vi "plot current.vi"() -> ()   [LabVIEW 2018]
uses:
  <vilib>/Utility/file.llb/Read Delimited Spreadsheet (string).vi
panel:
  out "Run, Subrun":i32[][](array[numeric])
  in  "Card.Channel":dbl=8.04
  in  "End":cluster{"Run":i32, "Subrun":i32}={"Run"=310, "Subrun"=-1}
  in  "Start":cluster{"Run":i32, "Subrun":i32}={"Run"=280, "Subrun"=0}
  out "Timestamp Array":timestamp[](array[timestamp])
  out "Plot":cluster{timestamp[], dbl[]}[](graph)
  # "channel must have 2 significant figures!"
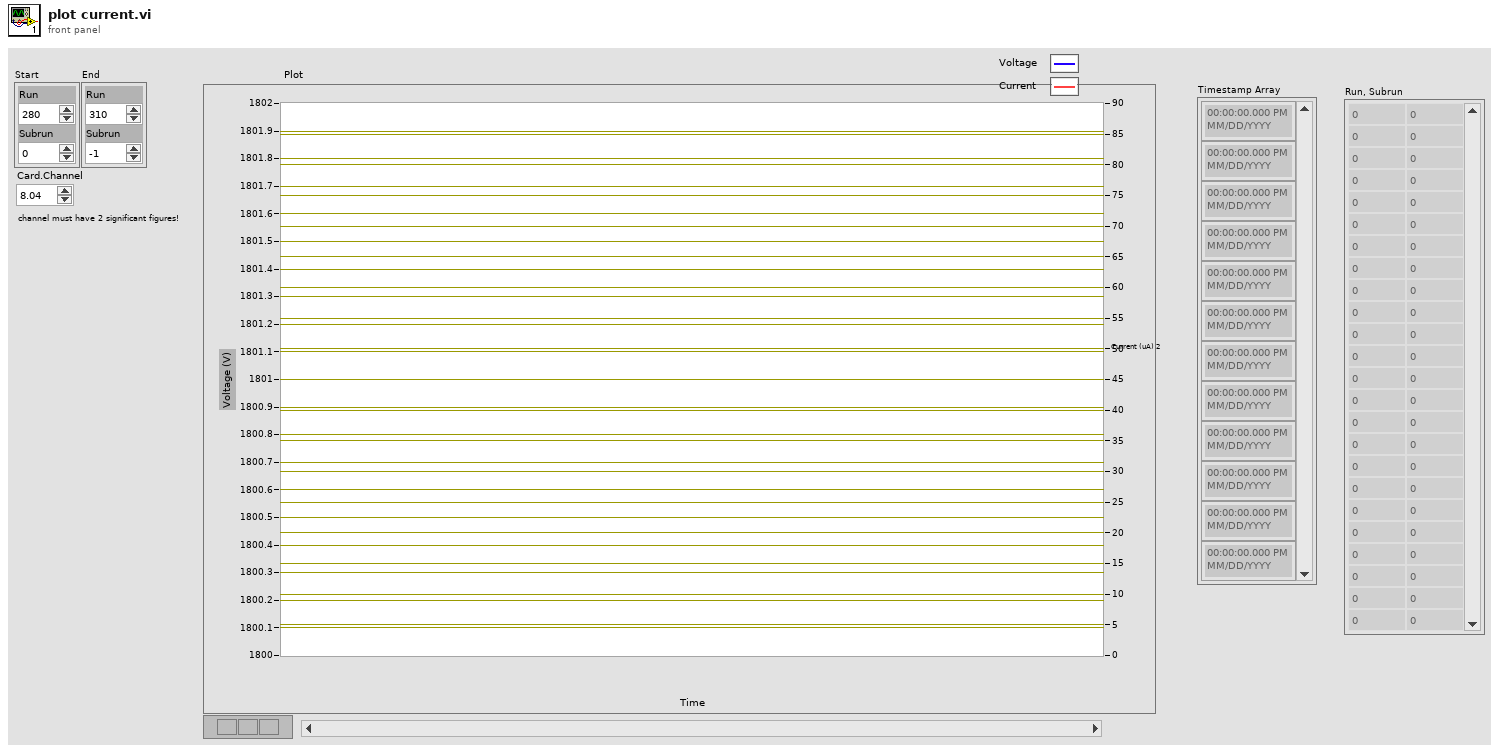
[diagram p1: front panel]
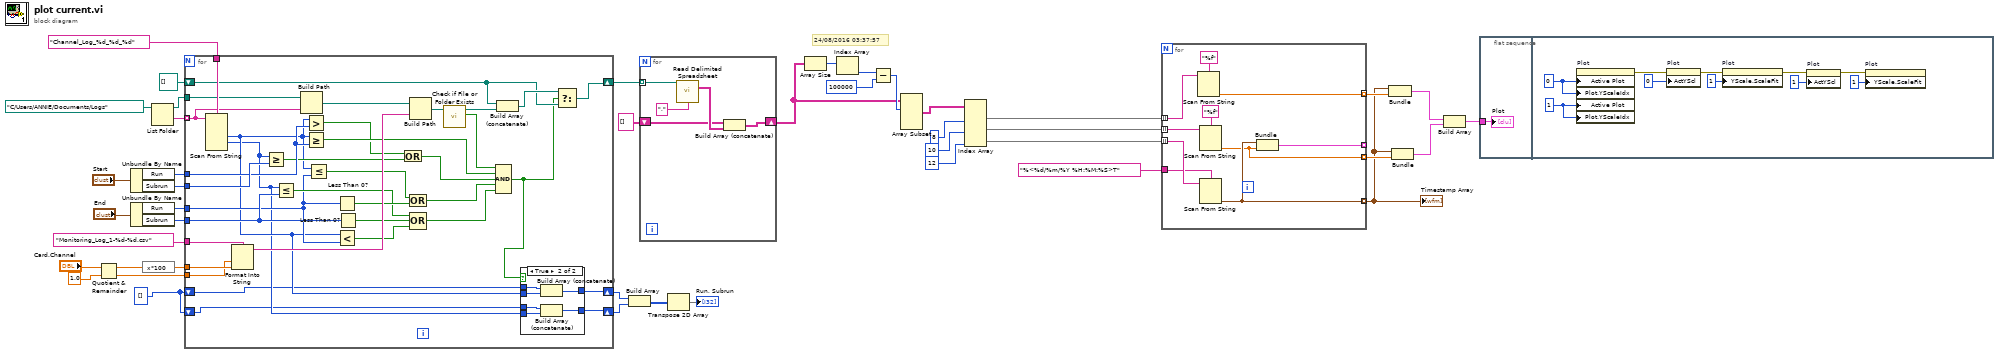
[diagram p0: block diagram]
diagram:
  w5 = i32[] []
  # "24/08/2016 03:37:57"
  n1 = Quotient & Remainder(x="Card.Channel", y=1.0) -> (x-y*floor(x/y)=w8:dbl, floor(x/y)=w12:dbl)
  n2 = Unbundle By Name("Start") -> ("Run"=w19:i32, "Subrun"=w18:i32)
  n3 = Unbundle By Name("End") -> ("Run"=w17:i32, "Subrun"=w16:i32)
  n4 = expression code="x*100"(w8) -> (w7:dbl)
  n5 = List Folder(path=path "C:/Users/ANNIE/Documents/Logs" ("file path (dialog if empty)")) -> (path out=w14:path, folder names=w24:string[])  [unwired: 3 in, 2 out]
  n6 = for {
    tunnel: w24 -> [w76] mode=indexing
    tunnel: w19 -> [w56]
    tunnel: w18 -> [w78]
    tunnel: w17 -> [w52]
    tunnel: w16 -> [w67]
    tunnel: "Channel_Log_%d_%d_%d" ("format string") -> [w79]
    shift-right: [w74] -> w10
    shift-left: path[] [] -> [w68]
    tunnel: w14 -> [w77]
    tunnel: w7 -> [w73]
    tunnel: w12 -> [w72]
    tunnel: "Monitoring_Log_1-%d-%d.csv" ("format string") -> [w71]
    shift-right: [w46] -> w3
    shift-left: w5 -> [w45]
    shift-right: [w47] -> w4
    shift-left: w5 -> [w44]
    n7 = Scan From String(format string=w79, input string=w76) -> (output 1=w49:i32, output 2=w48:i32)  [unwired: 6 in, 3 out]
    n8 = Format Into String(format string=w71, w72, w73) -> (resulting string=w70:string)  [unwired: 2 in, 1 out]
    n9 = Greater Or Equal?(x=w48, y=w78) -> (x >= y?=w54:bool)
    n10 = Less Or Equal?(x=w48, y=w67) -> (x <= y?=w64:bool)
    n11 = Build Path(base path=w77, name or relative path=w76) -> (appended path=w69:path)
    n12 = Greater?(x=w49, y=w56) -> (0:w55:bool)
    n13 = Greater Or Equal?(x=w49, y=w56) -> (x >= y?=w60:bool)
    n14 = Less Or Equal?(x=w49, y=w52) -> (x <= y?=w66:bool)
    n15 = Less Than 0?(x=w52) -> (x < 0?=w65:bool)
    n16 = Less?(x=w49, y=w52) -> (x < y?=w51:bool)
    n17 = Less Than 0?(x=w67) -> (x < 0?=w63:bool)
    n18 = Compound Arithmetic op=OR(w55, w54) -> (w53:bool)
    n19 = Build Path(base path=w69, name or relative path=w70) -> (appended path=w57:path)
    n20 = Compound Arithmetic op=OR(w66, w65) -> (w59:bool)
    n21 = Compound Arithmetic op=OR(w64, w63, w51) -> (w58:bool)
    n22 = call <vilib>:"Check if File or Folder Exists.vi"("path"=w57) -> ("file or folder exists?"=w61:bool, "dup path"=w62:path)  [unwired: 8 in, 1 out]
    n23 = Compound Arithmetic op=AND(w61, w60, w53, w59, w58) -> (w50:bool)
    n24 = Build Array (concatenate)(w68, w62) -> (w75:path[])
    n25 = case shown="True" w50 {
      tunnel: w49 -> [_ w87]
      tunnel: w48 -> [_ w86]
      tunnel: [w80 w85] -> w47
      tunnel: [w81 w84] -> w46
      tunnel: w45 -> [w81 w83]
      tunnel: w44 -> [w80 w82]
      frame False {
      }
      frame True {
        n26 = Build Array (concatenate)(w83, w87) -> (w84:i32[])
        n27 = Build Array (concatenate)(w82, w86) -> (w85:i32[])
      }
    }
    n28 = Select(t=w75, s=w50, f=w68) -> (s? t:f=w74:path[])
  }
  n29 = Build Array(w3, w4) -> (w2:i32[][])
  n30 = for {
    tunnel: w10 -> [w91] mode=indexing
    shift-right: [w89] -> w6
    shift-left: string[][] [] -> [w88]
    n31 = call-poly <vilib>:"Read Delimited Spreadsheet.vi"("file path (dialog if empty)"=w91, "delimiter (\\t)"="," ("delimiter (\\t)")) -> ("all rows"=w90:string[][])  [unwired: 8 in, 5 out]
    n32 = Build Array (concatenate)(w88, w90) -> (w89:string[][])
  }
  n33 = Transpose 2D Array(2D array=w2) -> (transposed array=→"Run, Subrun":i32[][])
  n34 = Array Size(array=w6) -> (size(s)=w43:i32[])
  n35 = Index Array(array=w43) -> (element=w42:i32)  [unwired: 1 in]
  n36 = Subtract(x=w42, y=100000 ("length")) -> (x-y=w40:i32)
  n37 = Array Subset(array=w6, index (row)=w40) -> (w39:string[][])  [unwired: 3 in]
  n38 = Index Array(array=w39, index (col) #1=8 ("length"), index (col) #2=10 ("length"), index (col) #3=12 ("length")) -> (element #1=w26:string[], element #2=w37:string[], element #3=w35:string[])  [unwired: 3 in]
  n39 = for {
    tunnel: w37 -> [w102] mode=indexing
    tunnel: w35 -> [w100] mode=indexing
    tunnel: "%<%d/%m/%Y %H:%M:%S>T" ("format string") -> [w99]
    tunnel: [w96] -> _ mode=indexing
    tunnel: [w98] -> w29 mode=indexing
    tunnel: [w95] -> w33 mode=indexing
    tunnel: [w94] -> w30 mode=indexing
    tunnel: w26 -> [w93] mode=indexing
    n40 = Scan From String(format string="%f", input string=w93) -> (output 1=w94:dbl)  [unwired: 3 in, 3 out]
    n41 = Scan From String(format string="%f", input string=w102) -> (output 1=w95:dbl)  [unwired: 3 in, 3 out]
    n42 = Scan From String(format string=w99, input string=w100) -> (output 1=w98:timestamp)  [unwired: 3 in, 3 out]
    n43 = Bundle(w98, w95) -> (w96:cluster{timestamp, dbl})  [unwired: 1 in]
  }
  "Timestamp Array" <- w29
  n44 = Bundle(w29, w30) -> (w28:cluster{timestamp[], dbl[]})  [unwired: 1 in]
  n45 = Bundle(w29, w33) -> (w32:cluster{timestamp[], dbl[]})  [unwired: 1 in]
  n46 = Build Array(w28, w32) -> (w31:cluster{timestamp[], dbl[]}[])
  n47 = flat-sequence {
    tunnel: w31 -> [w103]
    frame #0 {
      "Plot" <- w103
    }
    frame #1 {
      w112 = u32 1 ("Active Plot")
      w113 = u32 0 ("Active Plot")
      n48 = property on="Plot" class="XYGraph (strict)"("Active Plot"=w113, "Plot.YScaleIdx"=w113, "Active Plot"=w112, "Plot.YScaleIdx"=w112) -> (error out=w108:errorcluster)  [unwired: 2 in, 1 out]
      n49 = property on="Plot" class="XYGraph (strict)"(error in=w108, "ActYScl"=u8 0 ("Y Scale.Scale Fit")) -> (error out=w107:errorcluster)  [unwired: 1 in, 1 out]
      n50 = property on="Plot" class="XYGraph (strict)"(error in=w107, "YScale.ScaleFit"=u8 1 ("Y Scale.Scale Fit")) -> (error out=w105:errorcluster)  [unwired: 1 in, 1 out]
      n51 = property on="Plot" class="XYGraph (strict)"(error in=w105, "ActYScl"=u8 1 ("Y Scale.Scale Fit")) -> (error out=w104:errorcluster)  [unwired: 1 in, 1 out]
      n52 = property on="Plot" class="XYGraph (strict)"(error in=w104, "YScale.ScaleFit"=u8 1 ("Y Scale.Scale Fit")) -> ()  [unwired: 1 in, 2 out]
    }
  }
